vi "MacroOpsManager_MD.vi"() -> ()   [LabVIEW 2012]
doc: "SciScan 1.2 160622"
uses:
  HFG/Custom Controls and Typedefs/Heartbeat information cluster.ctl
  HFG/Custom Controls and Typedefs/Heartbeat Event Source.ctl
  Custom Controls/Heartbeat_States.ctl
  HFG/Custom Controls and Typedefs/HB_Error Conditions Cluster.ctl
  HFG/SubVIs/Master Slave messaging Flags.ctl
  HFG/Custom Controls and Typedefs/HB Actionable Event.ctl
  HFG/SubVIs/Heartbeat state manager Input VI names.ctl
  HFG/Custom Controls and Typedefs/HFG Commands.ctl
  Custom Controls/scan mode main settings tab.ctl
  image & display/Draw ROI on Line Scan Display Command.ctl
  Macro Rule/subVIs/MacroRules_FGV_Commands.ctl
  GFG/GFG library.lvlib
  handling front panel & ref & application control/Change GFG Boolean Control Property_Command.ctl
panel:
  out "Source VI":string
  out "String":string
  in  "Stop":bool
  out "Master-Slave messaging Flags":T1={"Instruction available"=TRUE, "Slave action completed"=TRUE, "Slave Ready?"=FALSE}
  out "Error conditions Cluster":T2
  out "Heartbeat information cluster":T3
  out "Master Instructions Issued":i32
  out "Slave Completions Received":i32
  out "Error Out":errorcluster
  in  "Error In":errorcluster
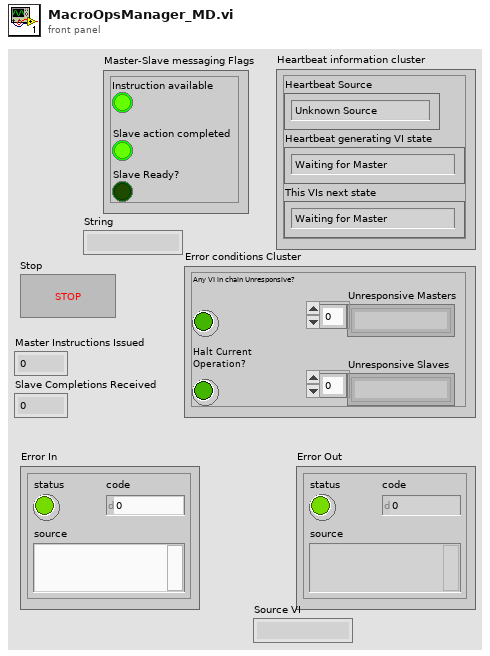
[diagram p1: front panel]
types:
  T1 = typedef "Master Slave messaging Flags.ctl" = cluster{"Instruction available":bool, "Slave action completed":bool, "Slave Ready?":bool}
  T2 = typedef "HB_Error Conditions Cluster.ctl" = cluster{"Any VI in chain Unresponsive?":bool, "Halt Current Operation?":bool, "Unresponsive Masters":string[], "Unresponsive Slaves":string[]}
  T3 = typedef "Heartbeat information cluster.ctl" = cluster{"Heartbeat Source":T4, "Heartbeat generating VI state":T5, "This VIs next state":T5}
  T4 = typedef "Heartbeat Event Source.ctl" = enum16{"Unknown Source", "Timeout", "This VI", "Master", "Slave"}
  T5 = typedef "Heartbeat_States.ctl" = enum16{"Waiting for Master", "Instruction Issued", "Waiting for Slave Completion", "Completed", "Cancelled", "Failed", "Broken Link"}
  T6 = typedef "Heartbeat state manager Input VI names.ctl" = cluster{"Current VI name":string, "Master VI Names":string[], "Slave VI Names":string[]}
  T7 = typedef "HB Actionable Event.ctl" = enum16{"Master instruction event", "Slave ready event", "Slave unavailable event", "Cancelled or Failed event", "Slave action complete event", "QUIT", "Broken Link", "Recovered from Broken Link"}
  T8 = typedef "HFG Commands.ctl" = enum16{"Set", "Get", "Initialize"}
  T9 = typedef "Draw ROI on Line Scan Display Command.ctl" = enum16{"Draw ROI from GFG", "Clear ROI"}
  T10 = typedef "scan mode main settings tab.ctl" = enum32{"2D frame", "2D line scan", "general settings", "Z Stack", "piezo"}
  T11 = typedef "MacroRules_FGV_Commands.ctl" = enum16{"Read File", "Get All", "Get Param and Flags"}
  T12 = cluster{"moveXabs":dbl, "moveYabs":dbl, "moveZabs":dbl}
  T13 = typedef "Macro_Action_List.ctl" = enum16{"Unknown Command", "2D.Frame.Scan", "2D.Line.Scan", "Load.Settings.File", "Move.To.Position", "Pause", "Z.Stack", "LOOP.Start", "LOOP.End", "Record", "Fast.Z", "Generic", "Slow.Z", "Tiling", "Preset.End"}
  T14 = cluster{"WaveformChartRef":refnum<vi>, "DigitalRef":refnum<vi>, "ArrayRef":refnum<vi>, "TabControlRef":refnum<vi>, "EnumRef":refnum<vi>, "RingRef":refnum<vi>, "BooleanRef":refnum<vi>, "KnobRef":refnum<vi>, "SlideRef":refnum<vi>, "PathRef":refnum<vi>, "StringRef":refnum<vi>, "ComboBox":refnum<vi>, "WaveformGraphRef":refnum<vi>}
  T15 = typedef "VariantType.lvlib/Type.ctl" = enum8{"Invalid Type", "Void", "I8", "I16", "I32", "I64", "U8", "U16", "U32", "U64", "Single Float", "Double Float", "Extended Float", "Single Complex", "Double Complex", "Extended Complex", "Enum U8", "Enum U16", "Enum U32", "Enum U64", "Single Float With Unit", "Double Float With Unit", "Extended Float With Unit", "Single Complex with Unit", "Double Complex with Unit", "Extended Complex with Unit", "Boolean", "String", "Path", "Picture", "Tag", "Array", "Cluster", "Variant", "LV Variant", "Waveform", "Timestamp", "Digital Waveform", "Digital Data", "ExpressData", "Refnum", "External Data", "VI", "Poly VI", "LabVIEW Class Instance", "Fixed Point"}
  T16 = typedef "Change GFG Boolean Control Property_Command.ctl" = enum16{"Enable", "Disable", "Disable and Grey", "Start Blinking", "Stop Blinking"}
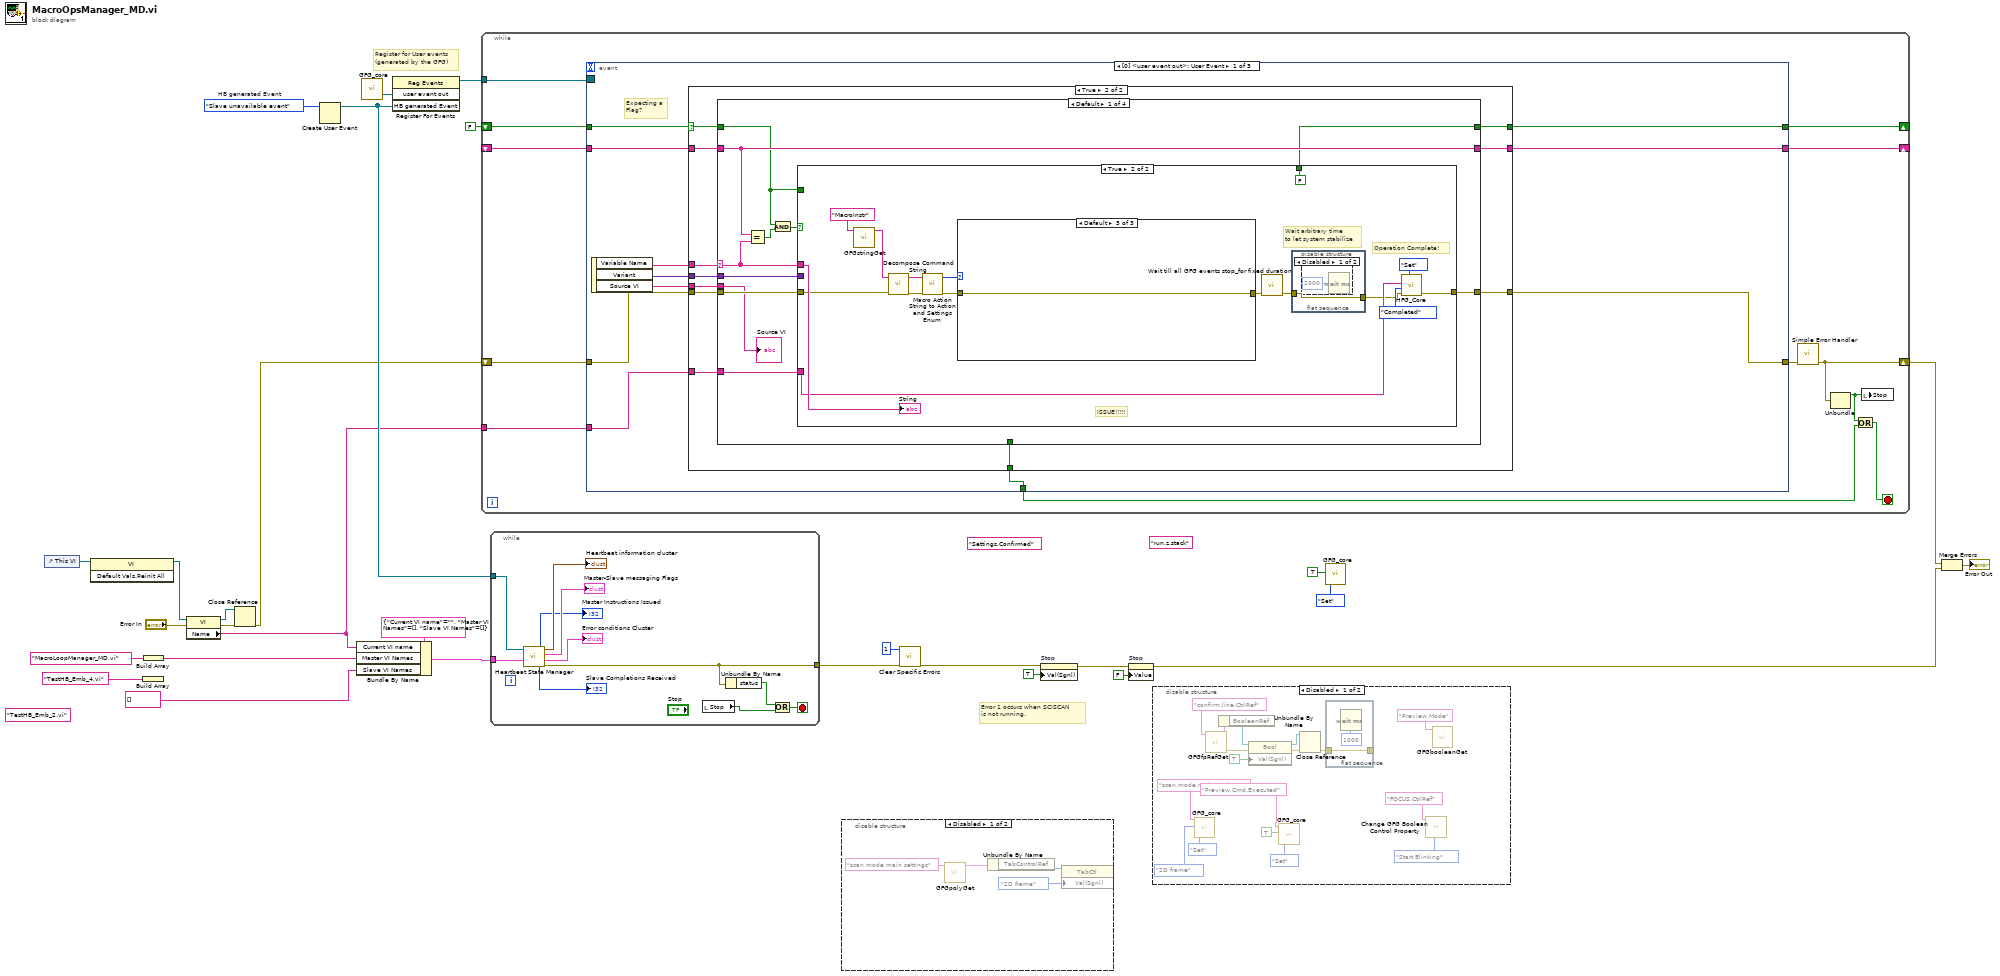
[diagram p0: block diagram]
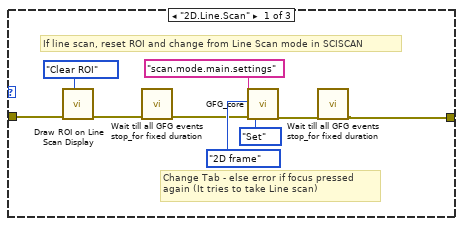
[diagram p7: hidden frame]
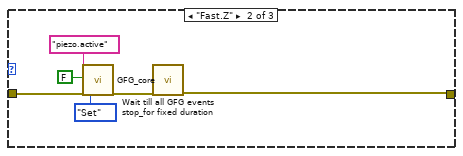
[diagram p8: hidden frame]
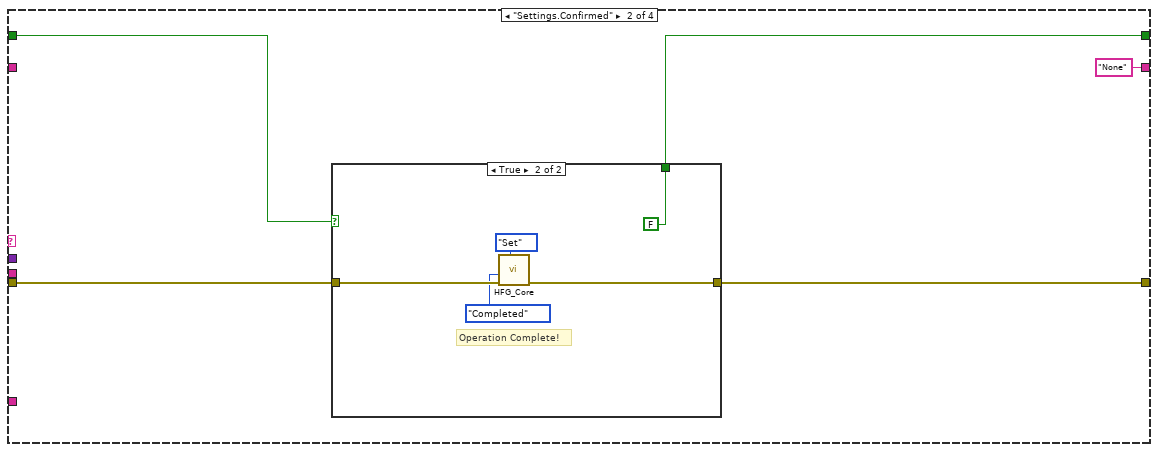
[diagram p9: hidden frame]
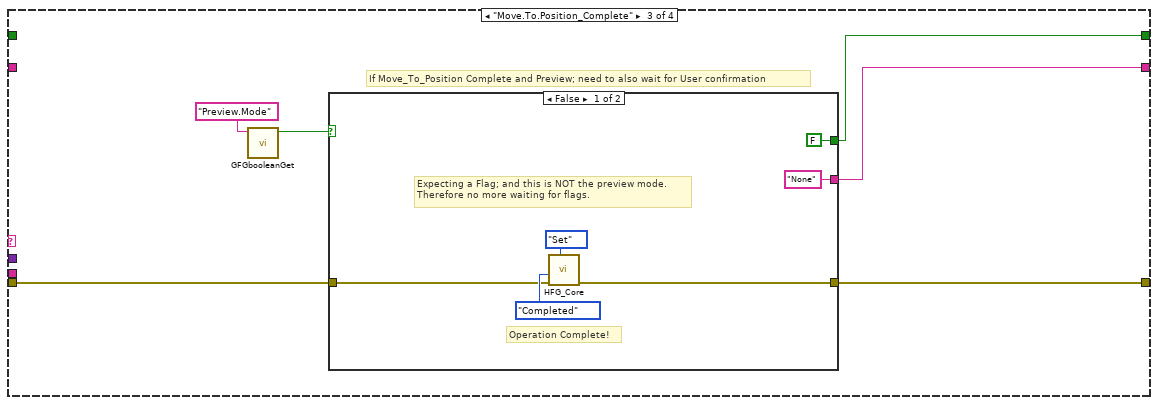
[diagram p11: hidden frame]
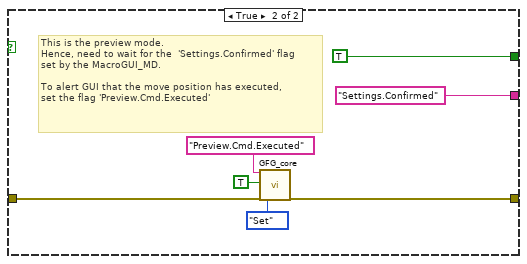
[diagram p12: hidden frame]
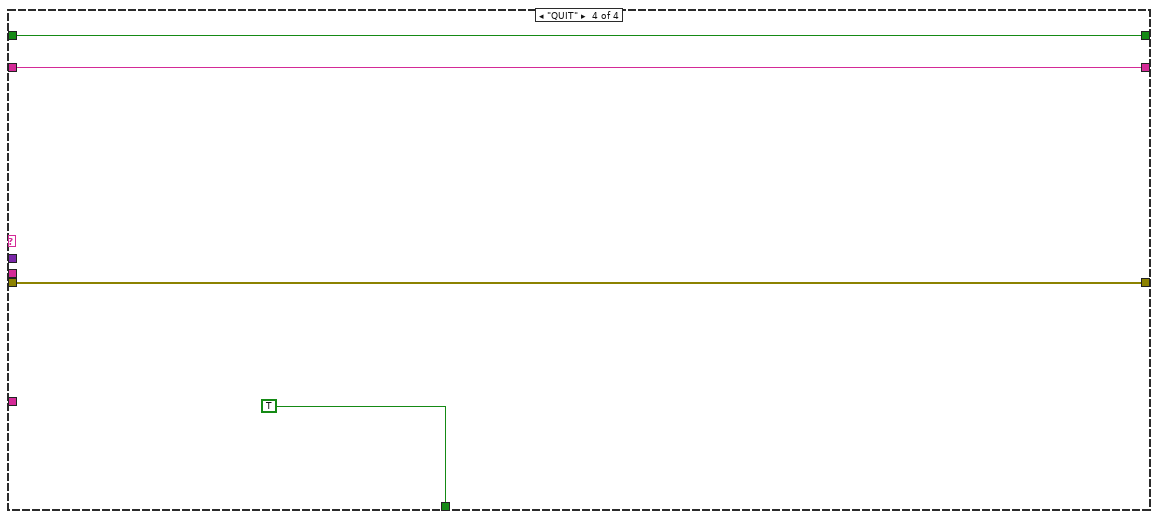
[diagram p13: hidden frame]
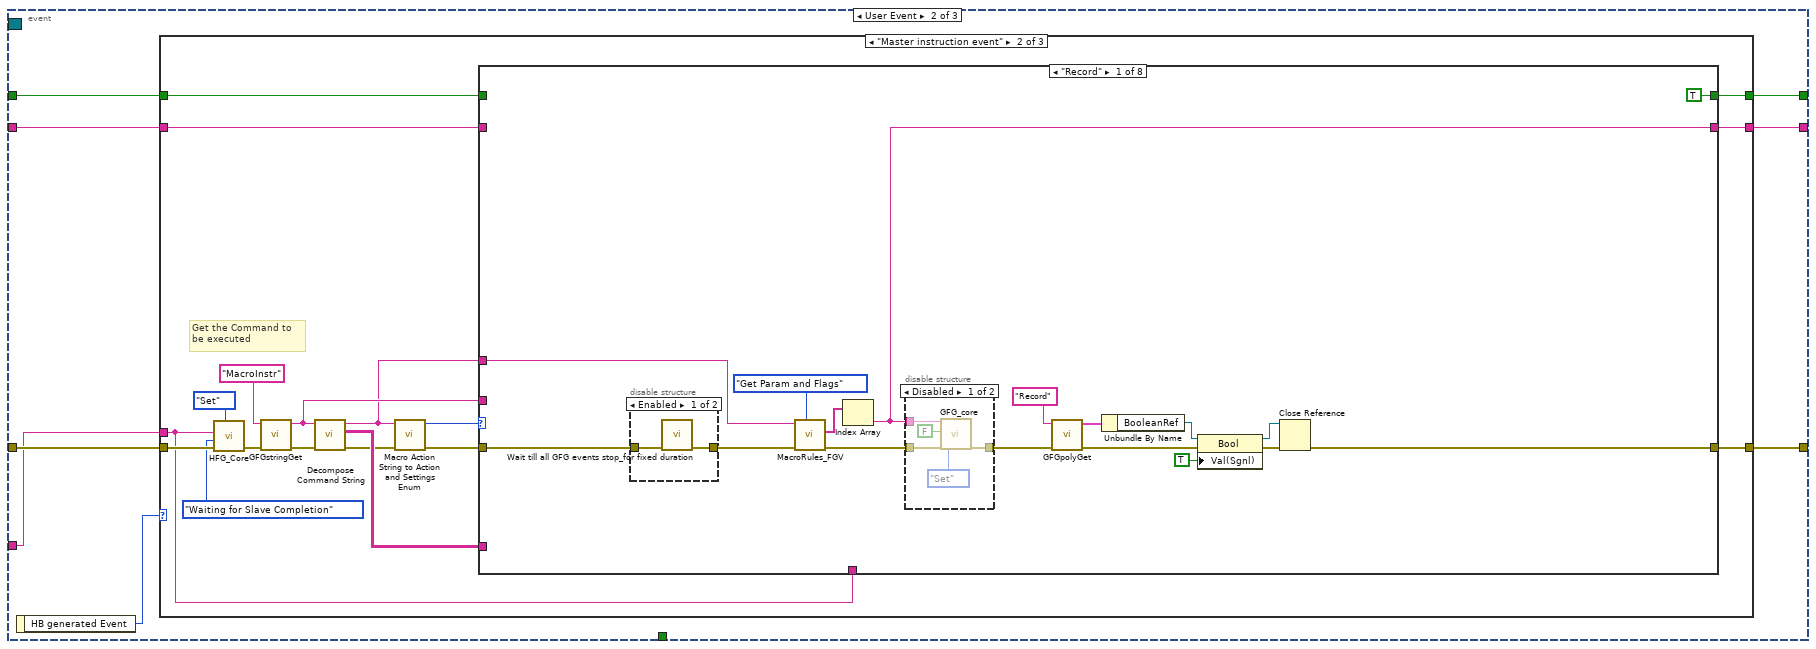
[diagram p14: hidden frame]
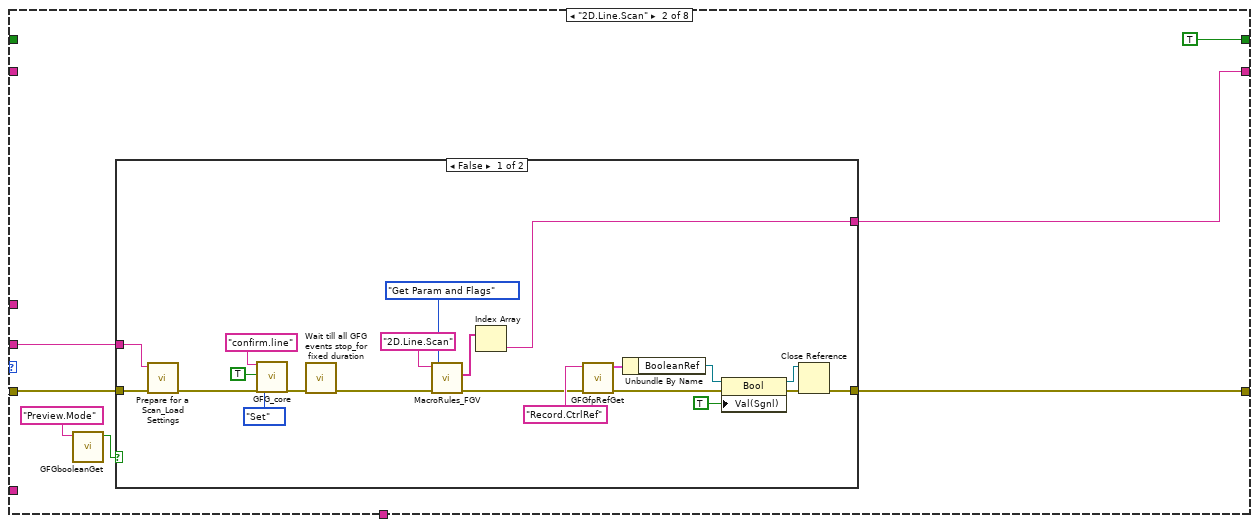
[diagram p18: hidden frame]
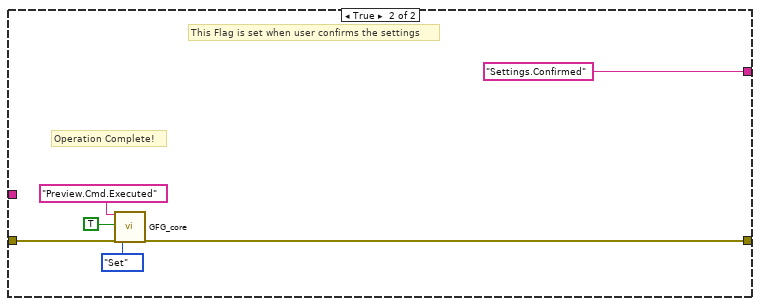
[diagram p19: hidden frame]
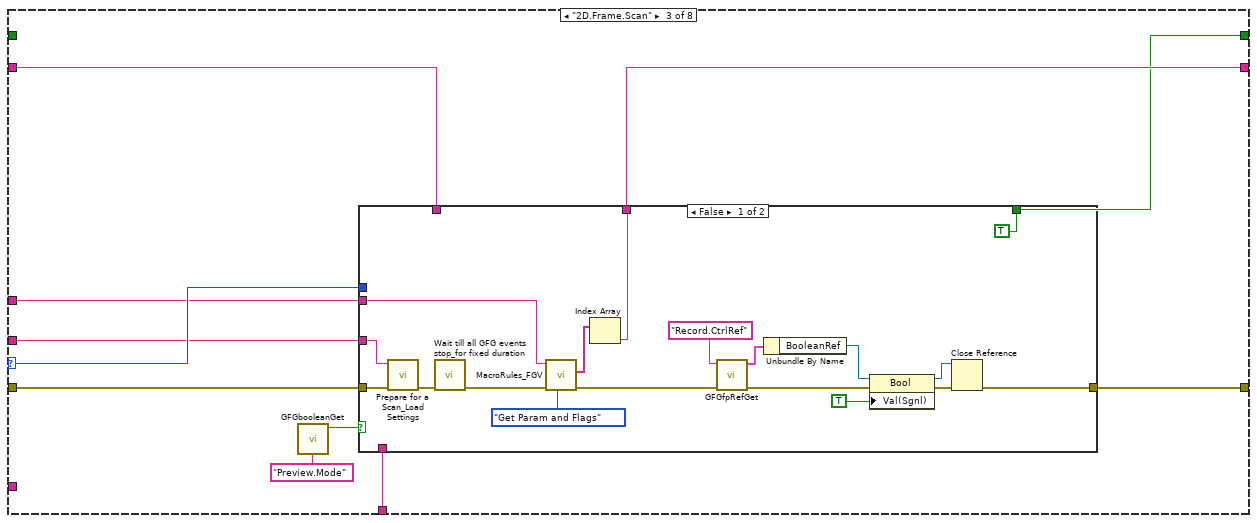
[diagram p20: hidden frame]
diagram:
  (unwired) "run.z.stack" ("Variable Name in")
  (unwired) "Settings.Confirmed"
  (unwired) "TestHB_Emb_2.vi"
  w27 = HB_Actionable_Event."Slave unavailable event"  # HB generated Event
  # "Error 1 occurs when SCISCAN\nis not running."
  # "Register for User events\n(generated by the GFG)"
  n1 = control-ref of="This VI"() -> (w9:refnum<vi>)
  n2 = invoke class="VI" method="Default Vals.Reinit All"(reference=w9) -> (reference out=w8:refnum<vi>)  [unwired: 2 in, 2 out]
  n3 = Build Array("TestHB_Emb_4.vi") -> ()  [unwired: 1 out]
  n4 = Build Array("MacroLoopManager_MD.vi") -> (w23:string[])
  n5 = property class="VI"(reference=w8, error in="Error In") -> (reference out=w6:refnum<vi>, error out=w7:errorcluster, "Name"=w19:string)
  n6 = Close Reference(reference=w6, error in (no error)=w7) -> (error out=w4:errorcluster)
  n7 = Create User Event(user event datatype=w27) -> (user event=w26:refnum<user-event>)  [unwired: 1 in, 1 out]
  n8 = Bundle By Name(cluster=T6 {"Current VI name"="", "Master VI Names"=[], "Slave VI Names"=[]} ("Heartbeat state manager Input VI names 2"), "Current VI name"=w19, "Master VI Names"=w23, "Slave VI Names"=string[] []) -> (w20:T6)
  n9 = call "GFG_core.vi"() -> ("user event out"=w29:refnum<user-event>)  [unwired: 13 in, 6 out]
  n10 = register-events(w29, w26) -> (reference out=w28:refnum<event-registration>)  [unwired: 2 in, 1 out]
  n11 = while {
    tunnel: w28 -> [w41]
    shift-right: [w39] -> _
    shift-left: _ -> [w38]
    shift-right: [w32] -> w11
    shift-left: w4 -> [w40]
    tunnel: w19 -> [w35]
    shift-right: [w31] -> _
    shift-left: FALSE -> [w30]
    stop <- w36 stop-if-true
    n12 = event shown="[0] <user event out>: User Event" {
      selector: w41 -> [_ _ _]
      dyn-events: _ -> [_ _ _]
      timeout: _ -> [_ _ _]
      tunnel: w40 -> [w51 w155 w443]
      tunnel: [w47 _ w442] -> w37
      tunnel: [w50 w156 w444] -> w39
      tunnel: w38 -> [w49 w152 w444]
      tunnel: [w48 w154 w443] -> w33
      tunnel: w35 -> [w44 w151 _]
      tunnel: [w45 w149 w441] -> w31
      tunnel: w30 -> [w43 w150 w441]
      event User Event {
        # "Expecting a\nFlag?"
        n13 = event-data() -> ("Variable Name"=w52:string, "Variant"=w46:variant, "Source VI"=w42:string)  [unwired: 1 in]
        n14 = case shown="True" w43 {
          selector: w43 -> [w53 w57]
          tunnel: w52 -> [_ w66]
          tunnel: w51 -> [w55 w65]
          tunnel: [w54 w64] -> w50
          tunnel: w49 -> [w54 w63]
          tunnel: [w55 w62] -> w48
          tunnel: [_ w61] -> w47
          tunnel: w46 -> [_ w60]
          tunnel: [w53 w59] -> w45
          tunnel: w44 -> [_ w58]
          tunnel: w42 -> [_ w56]
          frame False {
          }
          frame True {
            n15 = case shown="Default" w66 {
              selector: w66 -> [w76 _ _ _]
              tunnel: w65 -> [w74 w118 w129 w147]
              tunnel: [w77 "None" ("Variable Name in") w130 w148] -> w64
              tunnel: w63 -> [w77 _ _ w148]
              tunnel: [w73 w116 w128 w147] -> w62
              tunnel: [_ _ _ TRUE] -> w61
              tunnel: w60 -> [w75 _ _ _]
              tunnel: [w72 w114 w131 w145] -> w59
              tunnel: w57 -> [w68 w115 _ w145]
              tunnel: w58 -> [w71 _ _ _]
              tunnel: w56 -> [w67 _ _ _]
              frame Default {
                n16 = Equal?(x=w77, y=w76) -> (x = y?=w70:bool)
                n17 = And(x=w68, y=w70) -> (x .and. y?=w69:bool)
                n18 = case shown="True" w69 {
                  tunnel: w76 -> [_ w93]
                  tunnel: w75 -> [_ _]
                  tunnel: w74 -> [w79 w89]
                  tunnel: [w79 w95] -> w73
                  tunnel: [w78 FALSE] -> w72
                  tunnel: w71 -> [_ w92]
                  tunnel: w68 -> [w78 _]
                  frame False {
                  }
                  frame True {
                    # "Wait arbitrary time\nto let system stabilize"
                    # "ISSUE!!!!!"
                    # "Operation Complete!"
                    n19 = call "GFGstringGet.vi"("Variable Name in"="MacroInstr") -> ("String"=w86:string)  [unwired: 9 in, 1 out]
                    n20 = call "Decompose Command String.vi"("Error In"=w89, "Command IN"=w86) -> ("Error Out"=w85:errorcluster, "Action"=w83:string)  [unwired: 6 in, 2 out]
                    n21 = call "Macro Action String to Action and Settings Enum.vi"("error in (no error)"=w85, "Action String IN"=w83) -> ("error out"=w84:errorcluster, "Action Enum OUT"=w82:T13)  [unwired: 6 in, 2 out]
                    n22 = case shown="Default" w82 {
                      tunnel: w84 -> [w102 w108 w113]
                      tunnel: [w98 w107 w113] -> w88
                      frame "2D.Line.Scan" {
                        # "If line scan, reset ROI and change from Line Scan mode in SCISCAN"
                        # "Change Tab - else error if focus pressed again (It tries to take Line scan)"
                        n23 = call "Draw ROI on Line Scan Display.vi"("Draw ROI on Line Scan Display_Command"=Draw_ROI_on_Line_Scan_Display_Command."Clear ROI", "error in (no error)"=w102) -> ("error out"=w101:errorcluster)  [unwired: 9 in]
                        n24 = call "Wait till all GFG events stop_for fixed duration.vi"("error in (no error)"=w101) -> ("error out"=w99:errorcluster)  [unwired: 10 in]
                        n25 = call "GFG_core.vi"("Variable Name in"="scan.mode.main.settings", "Variant in"=scan_mode_main_settings_tab."2D frame" ("scan mode main settings"), "error in (no error)"=w99, "Action"=enum16{"Init", "Set", "Get"}."Set") -> ("error out"=w100:errorcluster)  [unwired: 9 in, 6 out]
                        n26 = call "Wait till all GFG events stop_for fixed duration.vi"("error in (no error)"=w100) -> ("error out"=w98:errorcluster)  [unwired: 10 in]
                      }
                      frame "Fast.Z" {
                        n27 = call "GFG_core.vi"("Variable Name in"="piezo.active", "Variant in"=FALSE, "error in (no error)"=w108, "Action"=enum16{"Init", "Set", "Get"}."Set") -> ("error out"=w110:errorcluster)  [unwired: 9 in, 6 out]
                        n28 = call "Wait till all GFG events stop_for fixed duration.vi"("error in (no error)"=w110) -> ("error out"=w107:errorcluster)  [unwired: 10 in]
                      }
                      frame Default {
                      }
                    }
                    n29 = call "Wait till all GFG events stop_for fixed duration.vi"("error in (no error)"=w88) -> ("error out"=w81:errorcluster)  [unwired: 10 in]
                    n30 = flat-sequence {
                      tunnel: w81 -> [w96]
                      tunnel: [w96] -> w80
                      frame #0 {
                        n31 = disable-structure shown="Disabled" {
                          frame Disabled {
                            n32 = Wait (ms)(milliseconds to wait=u32 2000) -> ()  [unwired: 1 out]
                          }
                          frame Enabled {
                          }
                        }
                      }
                    }
                    n33 = call "HFG_Core.vi"("HFG Commands"=HFG_Commands."Set", "Error In"=w80, "Heartbeat state IN"=Heartbeat_States."Completed", "VI Name (Calling VIs name by default)"=w92) -> ("Error Out"=w95:errorcluster)  [unwired: 4 in, 3 out]
                    "String" <- w93
                  }
                }
                "Source VI" <- w67
              }
              frame "Settings.Confirmed" {
                n34 = case shown="True" w115 {
                  selector: w115 -> [w120 _]
                  tunnel: w118 -> [w119 w125]
                  tunnel: [w119 w124] -> w116
                  tunnel: [w120 FALSE] -> w114
                  frame False {
                  }
                  frame True {
                    # "Operation Complete!"
                    n35 = call "HFG_Core.vi"("HFG Commands"=HFG_Commands."Set", "Error In"=w125, "Heartbeat state IN"=Heartbeat_States."Completed") -> ("Error Out"=w124:errorcluster)  [unwired: 5 in, 3 out]
                  }
                }
              }
              frame "Move.To.Position_Complete" {
                # "If Move_To_Position Complete and Preview; need to also wait for User confirmation"
                n36 = call "GFGbooleanGet.vi"("Variable Name in"="Preview.Mode") -> ("Boolean Value OUT"=w126:bool)  [unwired: 9 in, 1 out]
                n37 = case shown="False" w126 {
                  tunnel: [FALSE TRUE] -> w131
                  tunnel: ["None" ("Variable Name in") "Settings.Confirmed" ("Variable Name in")] -> w130
                  tunnel: w129 -> [w134 w140]
                  tunnel: [w133 w139] -> w128
                  frame False {
                    # "Operation Complete!"
                    # "Expecting a Flag; and this is NOT the preview mode.\nTherefore no more waiting for flags."
                    n38 = call "HFG_Core.vi"("HFG Commands"=HFG_Commands."Set", "Error In"=w134, "Heartbeat state IN"=Heartbeat_States."Completed") -> ("Error Out"=w133:errorcluster)  [unwired: 5 in, 3 out]
                  }
                  frame True {
                    # "This is the preview mode.\nHence, need to wait for the  'Settings.Confirmed' flag\nset by the MacroGUI_MD.\n\nTo alert GUI that the move position has executed, \nset the flag 'Preview.Cmd.Executed'"
                    n39 = call "GFG_core.vi"("Variable Name in"="Preview.Cmd.Executed", "Variant in"=TRUE, "error in (no error)"=w140, "Action"=enum16{"Init", "Set", "Get"}."Set") -> ("error out"=w139:errorcluster)  [unwired: 9 in, 6 out]
                  }
                }
              }
              frame "QUIT" {
              }
            }
          }
        }
      }
      event User Event {
        n40 = event-data() -> ("HB generated Event"=w153:T7)  [unwired: 1 in]
        n41 = case shown="\"Master instruction event\"" w153 {
          tunnel: [w159 w174 "None" ("Variable Name in")] -> w156
          tunnel: w155 -> [w158 w173 w439]
          tunnel: [w158 w172 w439] -> w154
          tunnel: w152 -> [w159 w171 _]
          tunnel: w151 -> [_ w168 _]
          tunnel: w150 -> [w157 w167 _]
          tunnel: [w157 w166 FALSE] -> w149
          frame Default {
          }
          frame "Master instruction event" {
            # "Get the Command to\nbe executed"
            n42 = call "HFG_Core.vi"("HFG Commands"=HFG_Commands."Set", "Heartbeat state IN"=Heartbeat_States."Waiting for Slave Completion", "VI Name (Calling VIs name by default)"=w168) -> ()  [unwired: 5 in, 4 out]
            n43 = call "GFGstringGet.vi"("Variable Name in"="MacroInstr" ("Source VI")) -> ("String"=w164:string)  [unwired: 9 in, 1 out]
            n44 = call "Decompose Command String.vi"("Error In"=w173, "Command IN"=w164) -> ("Error Out"=w163:errorcluster, "Parameter Table"=w175:string[][], "Action"=w160:string)  [unwired: 6 in, 1 out]
            n45 = call "Macro Action String to Action and Settings Enum.vi"("error in (no error)"=w163, "Action String IN"=w160) -> ("error out"=w162:errorcluster, "Action Enum OUT"=w161:T13)  [unwired: 6 in, 2 out]
            n46 = case shown="\"Record\"" w161 {
              selector: w161 -> [_ _ w242 _ _ _ _ _]
              tunnel: w175 -> [_ _ _ _ _ w356 _ w406]
              tunnel: w162 -> [w177 w203 w238 w273 w305 w355 w392 w405]
              tunnel: [w189 w208 w246 w280 w312 w357 "None" w401] -> w174
              tunnel: [w184 w205 w245 w279 w311 w350 w392 w400] -> w172
              tunnel: w171 -> [_ _ w241 w276 w308 w357 _ _]
              tunnel: w168 -> [_ _ w240 w275 w307 w352 _ _]
              tunnel: w167 -> [_ _ _ _ _ _ _ _]
              tunnel: [TRUE TRUE w239 w274 w306 FALSE FALSE TRUE] -> w166
              tunnel: w164 -> [_ w202 w237 w272 w304 _ _ _]
              tunnel: w160 -> [w178 _ w236 _ w303 _ _ w393]
              frame "Record" {
                n47 = disable-structure shown="Enabled" {
                  disable-tunnel: w177 -> [w200 w201]
                  disable-tunnel: [w199 w201] -> w176
                  frame Enabled {
                    n48 = call "Wait till all GFG events stop_for fixed duration.vi"("error in (no error)"=w200) -> ("error out"=w199:errorcluster)  [unwired: 10 in]
                  }
                  frame Disabled {
                  }
                }
                n49 = call "MacroRules_FGV.vi"("MacroRules_FGV_Commands"=MacroRules_FGV_Commands."Get Param and Flags", "Error In"=w176, "Command Name IN"=w178) -> ("Error Out"=w191:errorcluster, "Flags"=w190:string[])  [unwired: 4 in, 3 out]
                n50 = Index Array(array=w190) -> (element=w189:string)  [unwired: 1 in]
                n51 = disable-structure shown="Disabled" {
                  disable-tunnel: w191 -> [w196 w198]
                  disable-tunnel: w189 -> [w194 _]
                  disable-tunnel: [w193 w198] -> w182
                  frame Disabled {
                    n52 = call "GFG_core.vi"("Variable Name in"=w194, "Variant in"=FALSE, "error in (no error)"=w196, "Action"=enum16{"Init", "Set", "Get", "Clear"}."Set") -> ("error out"=w193:errorcluster)  [unwired: 9 in, 6 out]
                  }
                  frame Enabled {
                  }
                }
                n53 = call-poly "GFGpolyGet.vi"("error in (no error)"=w182, "Variable Name in"="Record") -> ("error out"=w180:errorcluster, "output cluster"=w181:T14)  [unwired: 8 in]
                n54 = Unbundle By Name(w181) -> ("BooleanRef"=w188:refnum<vi>)
                n55 = property class="Bool"(reference=w188, error in=w180, "Val(Sgnl)"=TRUE) -> (reference out=w185:refnum<vi>, error out=w186:errorcluster)
                n56 = Close Reference(reference=w185, error in (no error)=w186) -> (error out=w184:errorcluster)
              }
              frame "2D.Line.Scan" {
                n57 = call "GFGbooleanGet.vi"("Variable Name in"="Preview.Mode") -> ("Boolean Value OUT"=w206:bool)  [unwired: 9 in, 1 out]
                n58 = case shown="False" w206 {
                  tunnel: [w222 w233] -> w205
                  tunnel: [w218 "Settings.Confirmed"] -> w208
                  tunnel: w203 -> [w216 w235]
                  tunnel: w202 -> [w215 _]
                  frame False {
                    n59 = call "Prepare for a Scan_Load Settings.vi"("error in (no error)"=w216, "Command IN"=w215) -> ("error out"=w211:errorcluster)  [unwired: 9 in]
                    n60 = call "GFG_core.vi"("Variable Name in"="confirm.line", "Variant in"=TRUE, "error in (no error)"=w211, "Action"=enum16{"Init", "Set", "Get"}."Set") -> ("error out"=w209:errorcluster)  [unwired: 9 in, 6 out]
                    n61 = call "Wait till all GFG events stop_for fixed duration.vi"("error in (no error)"=w209) -> ("error out"=w214:errorcluster)  [unwired: 10 in]
                    n62 = call "MacroRules_FGV.vi"("MacroRules_FGV_Commands"=MacroRules_FGV_Commands."Get Param and Flags", "Error In"=w214, "Command Name IN"="2D.Line.Scan") -> ("Error Out"=w219:errorcluster, "Flags"=w221:string[])  [unwired: 4 in, 3 out]
                    n63 = Index Array(array=w221) -> (element=w218:string)  [unwired: 1 in]
                    n64 = call "GFGfpRefGet.vi"("error in (no error)"=w219, "Variable Name in"="Record.CtrlRef") -> ("error out"=w225:errorcluster, "output cluster"=w228:T14)  [unwired: 8 in]
                    n65 = Unbundle By Name(w228) -> ("BooleanRef"=w227:refnum<vi>)
                    n66 = property class="Bool"(reference=w227, error in=w225, "Val(Sgnl)"=TRUE) -> (reference out=w223:refnum<vi>, error out=w224:errorcluster)
                    n67 = Close Reference(reference=w223, error in (no error)=w224) -> (error out=w222:errorcluster)
                  }
                  frame True {
                    # "Operation Complete!"
                    # "This Flag is set when user confirms the settings"
                    n68 = call "GFG_core.vi"("Variable Name in"="Preview.Cmd.Executed", "Variant in"=TRUE, "error in (no error)"=w235, "Action"=enum16{"Init", "Set", "Get"}."Set") -> ("error out"=w233:errorcluster)  [unwired: 9 in, 6 out]
                  }
                }
              }
              frame "2D.Frame.Scan" {
                n69 = call "GFGbooleanGet.vi"("Variable Name in"="Preview.Mode") -> ("Boolean Value OUT"=w243:bool)  [unwired: 9 in, 1 out]
                n70 = case shown="False" w243 {
                  tunnel: w238 -> [w251 w266]
                  tunnel: [w252 "Settings.Confirmed" ("Variable Name in")] -> w246
                  tunnel: [w255 w265] -> w245
                  tunnel: w242 -> [_ _]
                  tunnel: w241 -> [_ _]
                  tunnel: w240 -> [_ _]
                  tunnel: [TRUE TRUE] -> w239
                  tunnel: w237 -> [w250 _]
                  tunnel: w236 -> [w247 _]
                  frame False {
                    n71 = call "Prepare for a Scan_Load Settings.vi"("error in (no error)"=w251, "Command IN"=w250) -> ("error out"=w249:errorcluster)  [unwired: 9 in]
                    n72 = call "Wait till all GFG events stop_for fixed duration.vi"("error in (no error)"=w249) -> ("error out"=w248:errorcluster)  [unwired: 10 in]
                    n73 = call "MacroRules_FGV.vi"("MacroRules_FGV_Commands"=MacroRules_FGV_Commands."Get Param and Flags", "Error In"=w248, "Command Name IN"=w247) -> ("Error Out"=w253:errorcluster, "Flags"=w263:string[])  [unwired: 4 in, 3 out]
                    n74 = Index Array(array=w263) -> (element=w252:string)  [unwired: 1 in]
                    n75 = call "GFGfpRefGet.vi"("error in (no error)"=w253, "Variable Name in"="Record.CtrlRef") -> ("error out"=w258:errorcluster, "output cluster"=w261:T14)  [unwired: 8 in]
                    n76 = Unbundle By Name(w261) -> ("BooleanRef"=w260:refnum<vi>)
                    n77 = property class="Bool"(reference=w260, error in=w258, "Val(Sgnl)"=TRUE) -> (reference out=w256:refnum<vi>, error out=w257:errorcluster)
                    n78 = Close Reference(reference=w256, error in (no error)=w257) -> (error out=w255:errorcluster)
                  }
                  frame True {
                    # "This is the preview mode. Set Flag to Indicate to the Macro GUI to prompt user for confirmation"
                    n79 = call "GFG_core.vi"("Variable Name in"="Preview.Cmd.Executed", "Variant in"=TRUE, "error in (no error)"=w266, "Action"=enum16{"Init", "Set", "Get"}."Set") -> ("error out"=w265:errorcluster)  [unwired: 9 in, 6 out]
                  }
                }
              }
              frame "Z.Stack" {
                # "This Case needs to be modified!!\n- Currently just a placeholder"
                n80 = call "GFGbooleanGet.vi"("Variable Name in"="Preview.Mode") -> ("Boolean Value OUT"=w277:bool)  [unwired: 9 in, 1 out]
                n81 = case shown="False" w277 {
                  tunnel: w273 -> [w286 w296]
                  tunnel: ["Scan_Complete" ("Variable Name in") "Settings.Confirmed"] -> w280
                  tunnel: [w290 w298] -> w279
                  tunnel: w276 -> [_ _]
                  tunnel: w275 -> [_ _]
                  tunnel: [TRUE TRUE] -> w274
                  tunnel: w272 -> [w285 _]
                  frame False {
                    # "This Variable is set to FALSE when Z.Stack run completed (in both Galco and Reso)"
                    n82 = call "Prepare for a Scan_Load Settings.vi"("error in (no error)"=w286, "Command IN"=w285) -> ("error out"=w284:errorcluster)  [unwired: 9 in]
                    n83 = call "Wait till all GFG events stop_for fixed duration.vi"("error in (no error)"=w284) -> ("error out"=w283:errorcluster)  [unwired: 10 in]
                    n84 = call "GFG_core.vi"("Variable Name in"="move.to.z.stack..start.plane", "Variant in"=TRUE, "error in (no error)"=w283, "Action"=enum16{"Init", "Set", "Get"}."Set") -> ("error out"=w282:errorcluster)  [unwired: 9 in, 6 out]
                    n85 = call "Wait till all GFG events stop_for fixed duration.vi"("error in (no error)"=w282) -> ("error out"=w281:errorcluster)  [unwired: 10 in]
                    n86 = call "GFG_core.vi"("Variable Name in"="start.z.stack", "Variant in"=TRUE, "error in (no error)"=w281, "Action"=enum16{"Init", "Set", "Get"}."Set") -> ("error out"=w290:errorcluster)  [unwired: 9 in, 6 out]
                  }
                  frame True {
                    # "This is the preview mode. No need to record!, and No flags"
                    n87 = call "GFG_core.vi"("Variable Name in"="Preview.Cmd.Executed", "Variant in"=TRUE, "error in (no error)"=w296, "Action"=enum16{"Init", "Set", "Get"}."Set") -> ("error out"=w298:errorcluster)  [unwired: 9 in, 6 out]
                  }
                }
              }
              frame "Fast.Z" {
                n88 = call "GFGbooleanGet.vi"("Variable Name in"="Preview.Mode") -> ("Boolean Value OUT"=w309:bool)  [unwired: 9 in, 1 out]
                n89 = case shown="False" w309 {
                  tunnel: w305 -> [w313 w344]
                  tunnel: [w330 "Settings.Confirmed"] -> w312
                  tunnel: [w319 w343] -> w311
                  tunnel: w308 -> [_ _]
                  tunnel: w307 -> [_ _]
                  tunnel: [TRUE TRUE] -> w306
                  tunnel: w304 -> [w335 _]
                  tunnel: w303 -> [w331 _]
                  frame False {
                    (unwired) "run.z.stack" ("Variable Name in")
                    # "This Variable is set to FALSE when Z.Stack run completed (in both Galco and Reso)"
                    n90 = call "Prepare for a Scan_Load Settings.vi"("error in (no error)"=w313, "Command IN"=w335) -> ("error out"=w334:errorcluster)  [unwired: 9 in]
                    n91 = call "Wait till all GFG events stop_for fixed duration.vi"("error in (no error)"=w334) -> ("error out"=w329:errorcluster)  [unwired: 10 in]
                    n92 = call "MacroRules_FGV.vi"("MacroRules_FGV_Commands"=MacroRules_FGV_Commands."Get Param and Flags", "Error In"=w329, "Command Name IN"=w331) -> ("Error Out"=w328:errorcluster, "Flags"=w332:string[])  [unwired: 4 in, 3 out]
                    n93 = Index Array(array=w332) -> (element=w330:string)  [unwired: 1 in]
                    n94 = disable-structure shown="Disabled" {
                      disable-tunnel: w328 -> [w338 _]
                      disable-tunnel: [w337 _] -> w315
                      frame Disabled {
                        n95 = call "GFG_core.vi"("Variable Name in"="move.to.z.stack..start.plane", "Variant in"=TRUE, "error in (no error)"=w338, "Action"=enum16{"Init", "Set", "Get"}."Set") -> ("error out"=w337:errorcluster)  [unwired: 9 in, 6 out]
                      }
                      frame Enabled {
                      }
                    }
                    n96 = call "GFG_core.vi"("Variable Name in"="piezo.active", "Variant in"=TRUE, "error in (no error)"=w315, "Action"=enum16{"Init", "Set", "Get"}."Set") -> ("error out"=w314:errorcluster)  [unwired: 9 in, 6 out]
                    n97 = call "Wait till all GFG events stop_for fixed duration.vi"("error in (no error)"=w314) -> ("error out"=w321:errorcluster)  [unwired: 10 in]
                    n98 = call-poly "GFGpolyGet.vi"("error in (no error)"=w321, "Variable Name in"="Record") -> ("error out"=w322:errorcluster, "output cluster"=w323:T14)  [unwired: 8 in]
                    n99 = Unbundle By Name(w323) -> ("BooleanRef"=w327:refnum<vi>)
                    n100 = property class="Bool"(reference=w327, error in=w322, "Val(Sgnl)"=TRUE) -> (reference out=w324:refnum<vi>, error out=w325:errorcluster)
                    n101 = Close Reference(reference=w324, error in (no error)=w325) -> (error out=w319:errorcluster)
                  }
                  frame True {
                    # "This is the preview mode. No need to record!, and No flags"
                    n102 = call "GFG_core.vi"("Variable Name in"="Preview.Cmd.Executed", "Variant in"=TRUE, "error in (no error)"=w344, "Action"=enum16{"Init", "Set", "Get"}."Set") -> ("error out"=w343:errorcluster)  [unwired: 9 in, 6 out]
                  }
                }
              }
              frame "Generic" {
                # "No flags for Generic command"
                n103 = for {
                  tunnel: w356 -> [w363] mode=indexing
                  shift-right: [w358] -> w351
                  shift-left: w355 -> [w358]
                  n104 = Index Array(array=w363) -> (element #1=w359:string, element #2=w360:string)  [unwired: 2 in]
                  n105 = call "GFG_core.vi"("Variable Name in"=w359, "Action"=enum16{"Init", "Set", "Get", "Clear"}."Get") -> ("Data Type Out"=w361:T15)  [unwired: 11 in, 6 out]
                  n106 = case shown="\"Boolean\"" w361 {
                    tunnel: w360 -> [_ w367 w375 w378 w383]
                    tunnel: w359 -> [_ w366 w369 w379 w386]
                    frame Default {
                    }
                    frame "I8".."Extended Complex" {
                      n107 = Fract/Exp String To Number(string=w367) -> (number=w364:dbl)  [unwired: 3 in, 1 out]
                      n108 = call "GFG_core.vi"("Variable Name in"=w366, "Variant in"=w364, "Action"=enum16{"Init", "Set", "Get", "Clear"}."Set") -> ()  [unwired: 10 in, 7 out]
                    }
                    frame "Boolean" {
                      n109 = To Upper Case(1:w375) -> (0:w376:string)
                      n110 = Equal?(x=w376, y="TRUE") -> (x = y?=w371:bool)
                      n111 = Select(t=TRUE, s=w371, f=FALSE) -> (s? t:f=w368:bool)
                      n112 = call "GFG_core.vi"("Variable Name in"=w369, "Variant in"=w368, "Action"=enum16{"Init", "Set", "Get", "Clear"}."Set") -> ()  [unwired: 10 in, 7 out]
                    }
                    frame "String" {
                      n113 = Search and Replace String(replace all?=TRUE ("replace all? (F)"), input string=w378, search string="'") -> (result string=w377:string)  [unwired: 5 in, 3 out]
                      n114 = call "GFG_core.vi"("Variable Name in"=w379, "Variant in"=w377, "Action"=enum16{"Init", "Set", "Get", "Clear"}."Set") -> ()  [unwired: 10 in, 7 out]
                    }
                    frame "Path" {
                      n115 = Search and Replace String(replace all?=TRUE ("replace all? (F)"), input string=w383, search string="'") -> (result string=w385:string)  [unwired: 5 in, 3 out]
                      n116 = String To Path(string=w385) -> (path=w384:path)
                      n117 = call "GFG_core.vi"("Variable Name in"=w386, "Variant in"=w384, "Action"=enum16{"Init", "Set", "Get", "Clear"}."Set") -> ()  [unwired: 10 in, 7 out]
                    }
                  }
                }
                n118 = call "HFG_Core.vi"("HFG Commands"=HFG_Commands."Set", "Error In"=w351, "Heartbeat state IN"=Heartbeat_States."Completed", "VI Name (Calling VIs name by default)"=w352) -> ("Error Out"=w350:errorcluster)  [unwired: 4 in, 3 out]
              }
              frame Default {
              }
              frame "Move.To.Position" {
                w417 = 1 ("disabled index (col)")
                n119 = Variant To Data(error in=w405, type=string[][] [], Variant=w406) -> (data=w421:string[][], error out=w399:errorcluster)
                n120 = Index Array(array=w421, index (row) #1=0 ("disabled index (row)"), index (col) #1=w417, index (row) #2=1 ("disabled index (row)"), index (col) #2=w417, index (row) #3=2 ("disabled index (row)"), index (col) #3=w417) -> (element #1=w416:string, element #2=w415:string, element #3=w414:string)
                n121 = Fract/Exp String To Number(string=w416) -> (number=w407:dbl)  [unwired: 3 in, 1 out]
                n122 = Fract/Exp String To Number(string=w415) -> (number=w408:dbl)  [unwired: 3 in, 1 out]
                n123 = Fract/Exp String To Number(string=w414) -> (number=w409:dbl)  [unwired: 3 in, 1 out]
                n124 = Bundle By Name(cluster=T12 {"moveXabs"=0.0, "moveYabs"=0.0, "moveZabs"=0.0} ("output cluster"), "moveXabs"=w407, "moveYabs"=w408, "moveZabs"=w409) -> (w410:T12)
                n125 = call "GFG_core.vi"("Variable Name in"="moveXYZabs", "Variant in"=w410, "error in (no error)"=w399, "Action"=enum16{"Init", "Set", "Get"}."Set") -> ("error out"=w398:errorcluster)  [unwired: 9 in, 6 out]
                n126 = call "MacroRules_FGV.vi"("MacroRules_FGV_Commands"=MacroRules_FGV_Commands."Get Param and Flags", "Error In"=w398, "Command Name IN"=w393) -> ("Error Out"=w403:errorcluster, "Flags"=w402:string[])  [unwired: 4 in, 3 out]
                n127 = Index Array(array=w402) -> (element=w401:string)  [unwired: 1 in]
                n128 = call "GFG_core.vi"("Variable Name in"="Initiate.Move_Flag", "Variant in"=TRUE, "error in (no error)"=w403, "Action"=enum16{"Init", "Set", "Get", "Clear"}."Set") -> ("error out"=w400:errorcluster)  [unwired: 9 in, 6 out]
              }
            }
          }
          frame "Cancelled or Failed event" {
            # "Stop stage first"
            # "Cancellation or Failure - Reset Flags;"
            n129 = call "GFG_core.vi"("Variable Name in"="Stage Stop", "Variant in"=TRUE, "Action"=enum16{"Init", "Set", "Get", "Clear"}."Set") -> ("error out"=w423:errorcluster)  [unwired: 10 in, 6 out]
            n130 = call "GFG_core.vi"("Variable Name in"="Shutter", "Variant in"=FALSE, "error in (no error)"=w423, "Action"=enum16{"Init", "Set", "Get", "Clear"}."Set") -> ("error out"=w428:errorcluster)  [unwired: 9 in, 6 out]
            n131 = call "GFG_core.vi"("Variable Name in"="Record", "Variant in"=FALSE, "error in (no error)"=w428, "Action"=enum16{"Init", "Set", "Get", "Clear"}."Set") -> ("error out"=w427:errorcluster)  [unwired: 9 in, 6 out]
            n132 = call "GFG_core.vi"("Variable Name in"="FOCUS", "Variant in"=FALSE, "error in (no error)"=w427, "Action"=enum16{"Init", "Set", "Get", "Clear"}."Set") -> ()  [unwired: 9 in, 7 out]
          }
        }
      }
      event "Stop": Value Change {
        n133 = event-data() -> ("NewVal"=w442:bool)  [unwired: 1 in]
      }
    }
    n134 = call <vilib>:"Simple Error Handler.vi"("error in (no error)"=w33) -> ("error out"=w32:errorcluster)  [unwired: 4 in, 4 out]
    n135 = Unbundle(w32) -> ("status"=w34:bool)  [unwired: 2 out]
    n136 = Or(x=w34, y=w37) -> (x .or. y?=w36:bool)
    n137 = local write "Stop"(w34) -> ()
  }
  n138 = while {
    tunnel: w20 -> [w455]
    tunnel: w26 -> [w451]
    tunnel: [w448] -> w17
    stop <- w446 stop-if-true
    n139 = call "Heartbeat State Manager.vi"("Heartbeat state manager Input VI names"=w455, "HB Command Event IN"=w451) -> ("Error Out"=w448:errorcluster, "Error conditions Cluster"=→"Error conditions Cluster":T2, "Master-Slave messaging Flags"=→"Master-Slave messaging Flags":T1, "Heartbeat information cluster"=→"Heartbeat information cluster":T3, "Slave Completions Received"=→"Slave Completions Received":i32, "Master Instructions Issued"=→"Master Instructions Issued":i32)  [unwired: 4 in]
    n140 = local read "Stop"() -> (w445:bool)
    n141 = Unbundle By Name(w448) -> ("status"=w447:bool)
    n142 = Or(x=w447, y=w445) -> (x .or. y?=w446:bool)
  }
  n143 = disable-structure shown="Disabled" {
    frame Disabled {
      n144 = call-poly "GFGpolyGet.vi"("Variable Name in"="scan mode main settings") -> ("output cluster"=w459:T14, "error in (no error)"=w460:errorcluster)  [unwired: 8 in, 1 out]
      n145 = Unbundle By Name(w459) -> ("TabControlRef"=w457:refnum<vi>)
      n146 = property class="TabCtl"(reference=w457, "Val(Sgnl)"=scan_mode_main_settings_tab."2D frame" ("scan mode main settings")) -> ()  [unwired: 1 in, 2 out]
    }
    frame Enabled {
    }
  }
  n147 = call "Clear Specific Errors.vi"("Error In"=w17, "Error number In"=1) -> ("Error Out"=w16:errorcluster)  [unwired: 8 in, 1 out]
  n148 = property on="Stop" class="Bool (strict)"(error in=w16, "Val(Sgnl)"=TRUE) -> (error out=w14:errorcluster)  [unwired: 1 in, 1 out]
  n149 = property on="Stop" class="Bool (strict)"(error in=w14, "Value"=FALSE) -> (error out=w10:errorcluster)  [unwired: 1 in, 1 out]
  n150 = disable-structure shown="Disabled" {
    frame Disabled {
      n151 = call "GFG_core.vi"("Variable Name in"="scan.mode.main.settings", "Variant in"=scan_mode_main_settings_tab."2D frame" ("scan mode main settings"), "Action"=enum16{"Init", "Set", "Get"}."Set") -> ()  [unwired: 10 in, 7 out]
      n152 = call "GFGfpRefGet.vi"("Variable Name in"="confirm.line.CtrlRef") -> ("error out"=w472:errorcluster, "output cluster"=w475:T14)  [unwired: 9 in]
      n153 = Unbundle By Name(w475) -> ("BooleanRef"=w474:refnum<vi>)
      n154 = property class="Bool"(reference=w474, error in=w472, "Val(Sgnl)"=TRUE) -> (reference out=w470:refnum<vi>, error out=w471:errorcluster)
      n155 = call "GFG_core.vi"("Variable Name in"="Preview.Cmd.Executed", "Variant in"=TRUE, "Action"=enum16{"Init", "Set", "Get"}."Set") -> ()  [unwired: 10 in, 7 out]
      n156 = Close Reference(reference=w470, error in (no error)=w471) -> (error out=w476:errorcluster)
      n157 = flat-sequence {
        tunnel: w476 -> [w480]
        tunnel: [w480] -> w477
        frame #0 {
          n158 = Wait (ms)(milliseconds to wait=u32 1000) -> ()  [unwired: 1 out]
        }
      }
      n159 = call "Change GFG Boolean Control Property.vi"("Change GFG Boolean Control Property_Command"=Change_GFG_Boolean_Control_Property_Command."Start Blinking", "GFG Boolean Control name IN (.CtrlRef)"="FOCUS.CtrlRef") -> ()  [unwired: 9 in, 1 out]
      n160 = call "GFGbooleanGet.vi"("Variable Name in"="Preview.Mode") -> ()  [unwired: 9 in, 2 out]
    }
    frame Enabled {
    }
  }
  n161 = call "GFG_core.vi"("Variant in"=TRUE, "Action"=enum16{"Init", "Set", "Get"}."Set") -> ()  [unwired: 11 in, 7 out]
  n162 = Merge Errors(w11, w10) -> (→"Error Out":errorcluster)
